vi "Slit_Positioner.vi"(0 "X pixel":dbl, 1 "Y pixel":dbl, 2 "X pixel":dbl, 3 "Y pixel":dbl, 4 "Serial (x) binning":dbl=1.0 min=1.0 step=1.0, 5 "Parallel (y) binning":dbl=1.0 min=1.0 step=1.0, 7 "Hour Angle (hrs)":dbl, 9 "Declination (deg)":dbl, 11 "Latitude (deg)":dbl=30.238, 13 "Parallactic Angle (deg)":dbl format="%#.3g") -> (14 "EW Offset":dbl caption="\"  to the" format="%#.2g", 15 "EW":u16(ring) items=["East", "West"], 16 "NS Offset":dbl caption="\"  to the" format="%#.2g", 17 "NS":u16(ring) items=["North", "South"])   [LabVIEW 2015]
panel:
  in  "Compute Parallactic Angle?":bool
  # "Goodman Spectrograph Slit Alignment Tool"
  # "Parallactic Angle"
  # "Binning"
  # "Required SOAR Telescope Offset"
  # "Slit Coordinates"
  # "Object Coord."
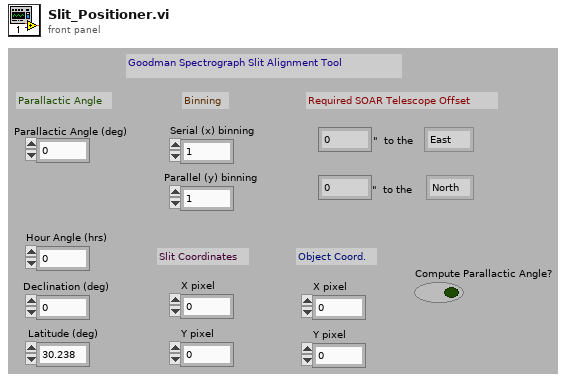
[diagram p1: front panel]
types:
  T1 = cluster{"Latitude (deg)":dbl, "Declination (deg)":dbl}
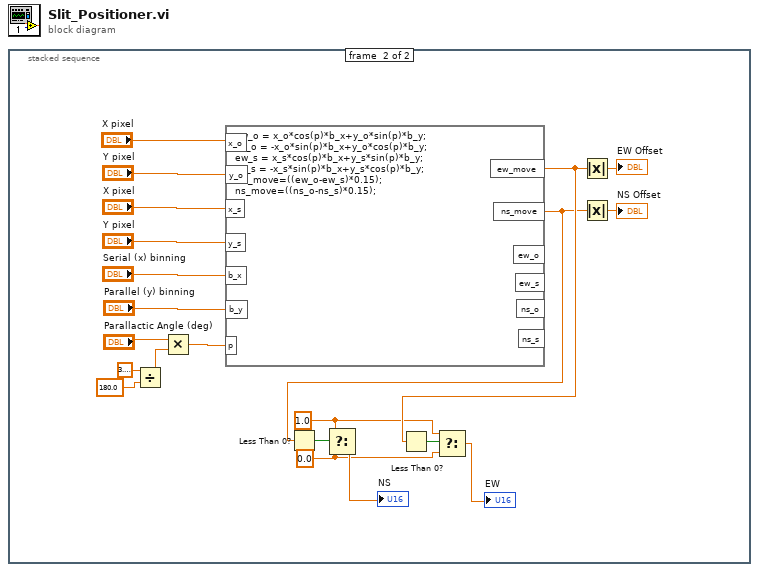
[diagram p0: block diagram]
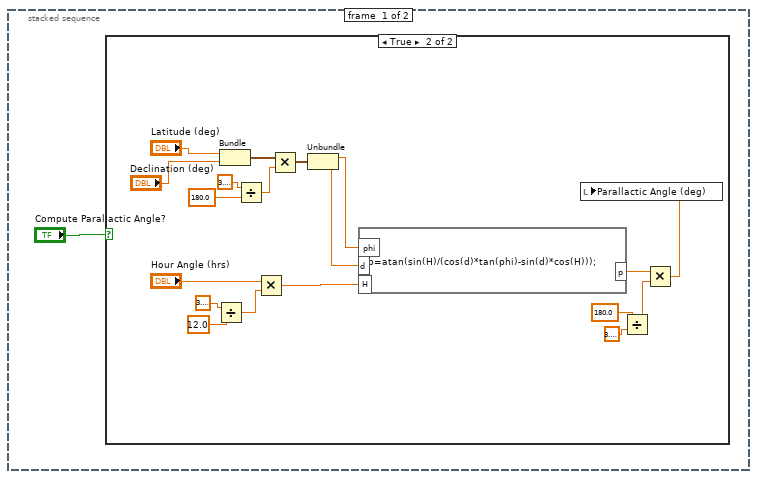
[diagram p2: hidden frame]
diagram:
  n1 = stacked-sequence {
    frame #0 {
      n2 = case shown="True" "Compute Parallactic Angle?" {
        frame False {
        }
        frame True {
          n3 = Divide(x=3.141592653589793, y=12.0) -> (x/y=w10:dbl)
          n4 = Bundle("Latitude (deg)"="Latitude (deg)", "Declination (deg)"="Declination (deg)") -> (w4:T1)  [unwired: 1 in]
          n5 = Divide(x=3.141592653589793, y=180.0) -> (x/y=w7:dbl)
          n6 = Multiply(x="Hour Angle (hrs)", y=w10) -> (x*y=w15:dbl)
          n7 = Multiply(x=w4, y=w7) -> (x*y=w8:T1)
          n8 = Unbundle(w8) -> ("Latitude (deg)"=w13:dbl, "Declination (deg)"=w14:dbl)
          n9 = formula code="p=atan(sin(H)/(cos(d)*tan(phi)-sin(d)*cos(H)));"("H"=w15, "d"=w14, "phi"=w13) -> ("p"=w16:dbl)
          n10 = Divide(x=180.0, y=3.141592653589793) -> (x/y=w19:dbl)
          n11 = Multiply(x=w16, y=w19) -> (x*y=w20:dbl)
          n12 = local write "Parallactic Angle (deg)"(w20) -> ()
        }
      }
    }
    frame #1 {
      w29 = 0.0 ("f")
      w28 = 1.0 ("t")
      n13 = Divide(x=3.141592653589793, y=180.0) -> (x/y=w39:dbl)
      n14 = Multiply(x="Parallactic Angle (deg)", y=w39) -> (x*y=w41:dbl)
      n15 = formula code="ew_o = x_o*cos(p)*b_x+y_o*sin(p)*b_y;\nns_o = -x_o*sin(p)*b_x+y_o*cos(p)*b_y;\new_s = x_s*cos(p)*b_x+y_s*sin(p)*b_y;\nns_s = -x_s*sin(p)*b_x+y_s*cos(p)*b_y;\new_move=((ew_o-ew_s)*0.15);\nns_move=((ns_o-ns_s)*0.15);"("x_o"="X pixel", "y_o"="Y pixel", "x_s"="X pixel", "y_s"="Y pixel", "b_x"="Serial (x) binning", "b_y"="Parallel (y) binning", "p"=w41) -> ("ew_move"=w35:dbl, "ns_move"=w33:dbl)  [unwired: 4 out]
      n16 = Less Than 0?(x=w33) -> (x < 0?=w27:bool)
      n17 = Select(t=w28, s=w27, f=w29) -> (s? t:f=→"NS":dbl)
      n18 = Less Than 0?(x=w35) -> (x < 0?=w30:bool)
      n19 = Select(t=w28, s=w30, f=w29) -> (s? t:f=→"EW":dbl)
      n20 = Absolute Value(x=w35) -> (abs(x)=→"EW Offset":dbl)
      n21 = Absolute Value(x=w33) -> (abs(x)=→"NS Offset":dbl)
    }
  }
